vi "BRig_dataBlock_c_nTimeout_total_R.vi"() -> (2 "output_c_nTimeout_total_R":i32)   [LabVIEW 2014]
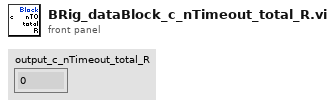
[diagram p1: front panel]
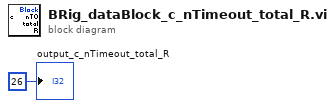
[diagram p0: block diagram]
diagram:
  "output_c_nTimeout_total_R" <- 26 ("output_iBlock")
